vi "create public folders.vi"(8 "error in":errorcluster) -> (0 "error out":errorcluster)   [LabVIEW 2020]
uses:
  <vilib>/Utility/sysdir.llb/System Directory Type.ctl
panel:
  out "Array":path[](array[path])
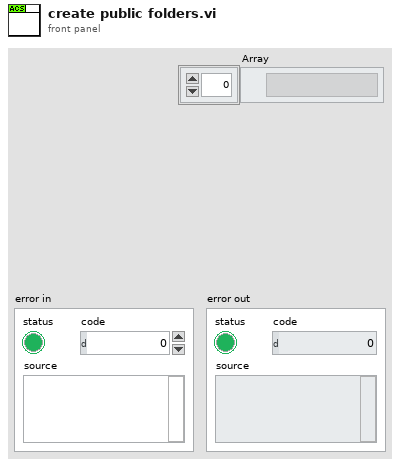
[diagram p1: front panel]
types:
  T1 = typedef "System Directory Type.ctl" = i32
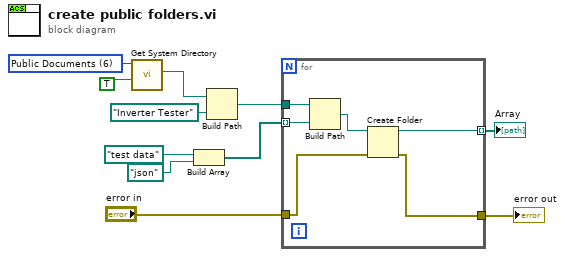
[diagram p0: block diagram]
diagram:
  w11 = T1 6 items=["User Home"=0, "User Desktop"=1, "User Documents"=2, "User Application Data"=3, "User Preferences"=4, "User Temporary"=5, "Public Documents"=6, "Public Application Data"=7, "Public Preferences"=8, "Public Cache"=13, "System Core Libraries"=9, "System Installed Libraries"=10, "Application Files"=11, "Boot Volume Root"=12] ("system directory type")
  n1 = call <vilib>:"Get System Directory.vi"("create directory if not found? (F)"=TRUE, "system directory type"=w11) -> ("system directory"=w10:path)  [unwired: 9 in]
  n2 = Build Array(path "test data" ("name or relative path"), path "json" ("name or relative path")) -> (w4:path[])
  n3 = Build Path(base path=w10, name or relative path=path "Inverter Tester") -> (appended path=w5:path)
  n4 = for {
    tunnel: w5 -> [w17]
    tunnel: w4 -> [w16] mode=indexing
    tunnel: [w14] -> w3 mode=indexing
    tunnel: "error in" -> [w13]
    tunnel: [w12] -> w1
    n5 = Build Path(base path=w17, name or relative path=w16) -> (appended path=w15:path)
    n6 = Create Folder(path (use dialog)=w15, error in=w13) -> (created path=w14:path, error out=w12:errorcluster)  [unwired: 1 in, 1 out]
  }
  "error out" <- w1
  "Array" <- w3
